vi "Launch Asynchronous Execution Units.vi"(8 "error in":errorcluster, 10 "RTStateVariables in":T2 {"Inline Execution Units"."Outgoing Data References"."Data Reference" format="%.0x"; "Inline Execution Units"."Incoming Data References" format="%.0x"}, 11 "Device Ref in":T1 format="%.0x") -> (0 "error out":errorcluster, 2 "RTStateVariables out":T2 {"Inline Execution Units"."Outgoing Data References"."Data Reference" format="%.0x"; "Inline Execution Units"."Incoming Data References" format="%.0x"}, 3 "Device Ref out":T1 format="%.0x")   [LabVIEW 2020, in "Ballard ARINC 429 Engine.lvlib" / "Custom Device.lvlib"]
uses:
  Custom Device.lvlib
  RTStateVariables.ctl
  <vilib>/NI/NIVS Inline Async API/_VS Inline Async API/VS Inline Async API/VS Inline Async API.lvclass
  Interfaces/Shared Resources/Shared Resources.lvclass
  Inline Execution Unit Runtime Information.ctl
  Interfaces/Execution Unit/Execution Unit.lvclass
  <vilib>/NI VeriStand/Custom Device API/Data Reference.ctl
  <vilib>/NI VeriStand/Custom Device API/Block Data Reference.ctl
  Asynchronous Execution Unit Runtime Information.ctl
  <vilib>/NI VeriStand/Custom Device API/Custom Device Item Ref.ctl
  Asynchronous Process Parameters.ctl
  <vilib>/NI VeriStand/Custom Device API/Custom Device API.lvlib
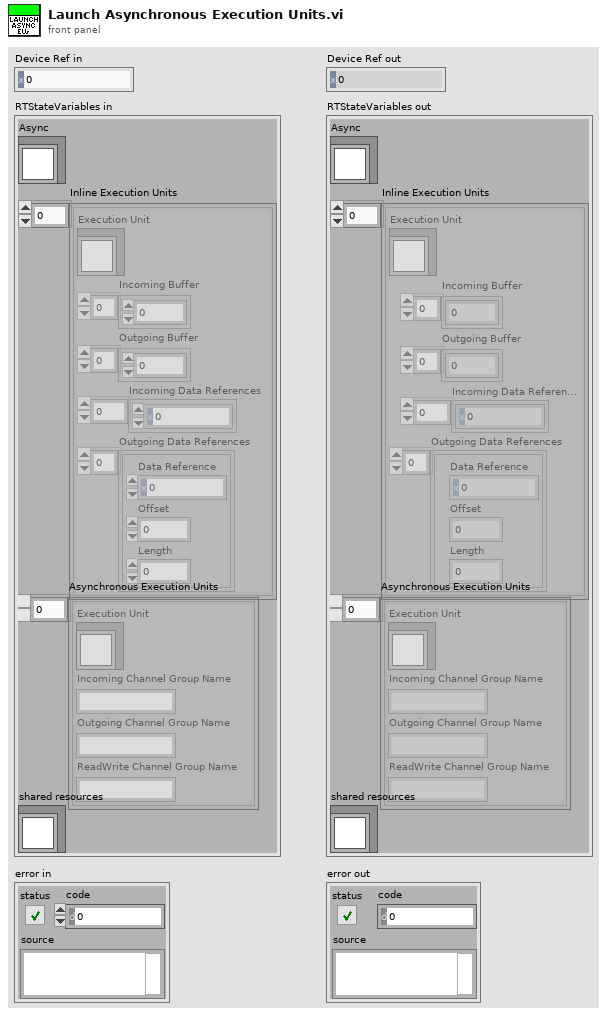
[diagram p1: front panel]
types:
  T1 = typedef "Custom Device API.lvlib/Custom Device Item Ref.ctl" = u64
  T2 = typedef "Ballard ARINC 429 Engine.lvlib/Custom Device.lvlib/RTStateVariables.ctl" = cluster{"Async":refnum<class "VS Inline Async API.lvclass">, "Inline Execution Units":T3[], "Asynchronous Execution Units":T6[], "shared resources":refnum<class "Shared Resources.lvclass">}
  T3 = typedef "Ballard ARINC 429 Engine.lvlib/Custom Device.lvlib/Inline Execution Unit Runtime Information.ctl" = cluster{"Execution Unit":refnum<class "Execution Unit.lvclass">, "Incoming Buffer":dbl[], "Outgoing Buffer":dbl[], "Incoming Data References":T4[], "Outgoing Data References":T5[]}
  T4 = typedef "Custom Device API.lvlib/Data Reference.ctl" = i32
  T5 = typedef "Custom Device API.lvlib/Block Data Reference.ctl" = cluster{"Data Reference":T4, "Offset":u64, "Length":u64}
  T6 = typedef "Ballard ARINC 429 Engine.lvlib/Custom Device.lvlib/Asynchronous Execution Unit Runtime Information.ctl" = cluster{"Execution Unit":refnum<class "Execution Unit.lvclass">, "Incoming Channel Group Name":string, "Outgoing Channel Group Name":string, "ReadWrite Channel Group Name":string}
  T7 = typedef "Asynchronous Process Parameters.ctl" = cluster{"Asynchronous Execution Unit Runtime Information":T6, "shared resources":refnum<class "Shared Resources.lvclass">}
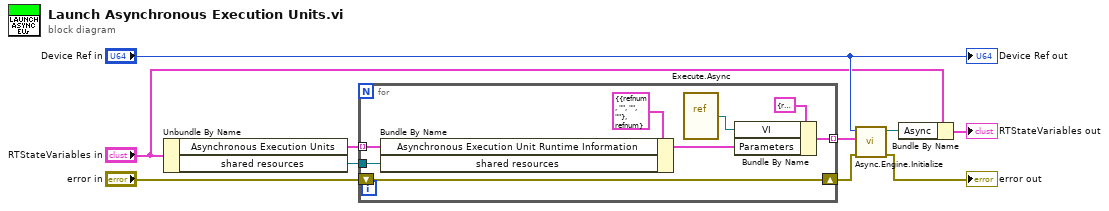
[diagram p0: block diagram]
diagram:
  n1 = Unbundle By Name("RTStateVariables in") -> ("Asynchronous Execution Units"=w5:T6[], "shared resources"=w2:refnum<class "Shared Resources.lvclass">)
  n2 = for {
    tunnel: w5 -> [w14] mode=indexing
    tunnel: [w17] -> w4 mode=indexing
    shift-right: [w15] -> w1
    shift-left: "error in" -> [w15]
    tunnel: w2 -> [w13]
    n3 = Bundle By Name(cluster=T7 {"Asynchronous Execution Unit Runtime Information"={"Execution Unit"=refnum, "Incoming Channel Group Name"="", "Outgoing Channel Group Name"="", "ReadWrite Channel Group Name"=""}, "shared resources"=refnum}, "Asynchronous Execution Unit Runtime Information"=w14, "shared resources"=w13) -> (w11:T7)
    n4 = vi-ref "Execute.Async.vi"() -> (w16:refnum<vi>)
    n5 = Bundle By Name(cluster=cluster{"VI":refnum<vi>, "Parameters":variant} {"VI"=refnum, "Parameters"=variant} ("Process"), "VI"=w16, "Parameters"=w11) -> (w17:cluster{"VI":refnum<vi>, "Parameters":variant})
  }
  n6 = call <vilib>:"Async.Engine.Initialize.vi"("error in (no error)"=w1, "Processes"=w4, "Custom Device Ref"="Device Ref in") -> ("error out"=→"error out":errorcluster, "Async"=w7:refnum<class "VS Inline Async API.lvclass">)  [unwired: 7 in]
  n7 = Bundle By Name(cluster="RTStateVariables in", "Async"=w7) -> (→"RTStateVariables out":T2)
  "Device Ref out" <- "Device Ref in"
